vi "sub vi - temperature delay v2.vi"(10 "temp values IN":T1, 11 "temp signals":T2) -> (0 "T2-N":dbl, 1 "T2-L":dbl, 2 "T1-N":dbl, 3 "T1-L":dbl, 4 "temp values OUT":T1)   [LabVIEW 2013]
uses:
  program files/Global 1.vi
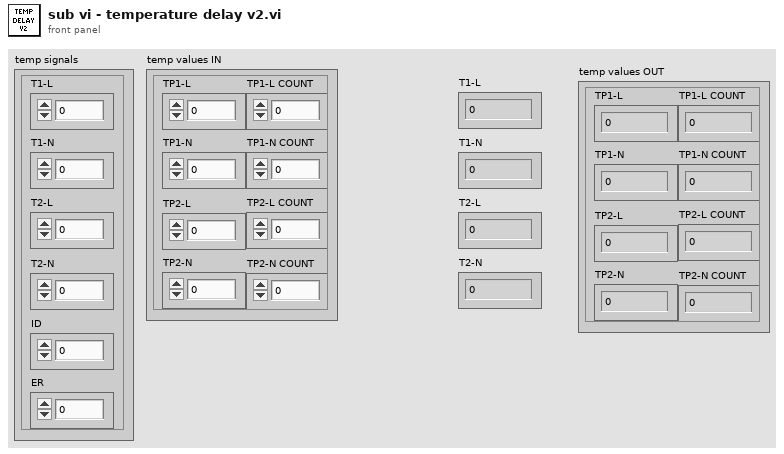
[diagram p1: front panel]
types:
  T1 = cluster{"TP1-L":dbl, "TP1-N":dbl, "TP2-L":dbl, "TP2-N":dbl, "TP1-L COUNT":dbl, "TP1-N COUNT":dbl, "TP2-L COUNT":dbl, "TP2-N COUNT":dbl}
  T2 = cluster{"T1-L":dbl, "T1-N":dbl, "T2-L":dbl, "T2-N":dbl, "ID":dbl, "ER":dbl}
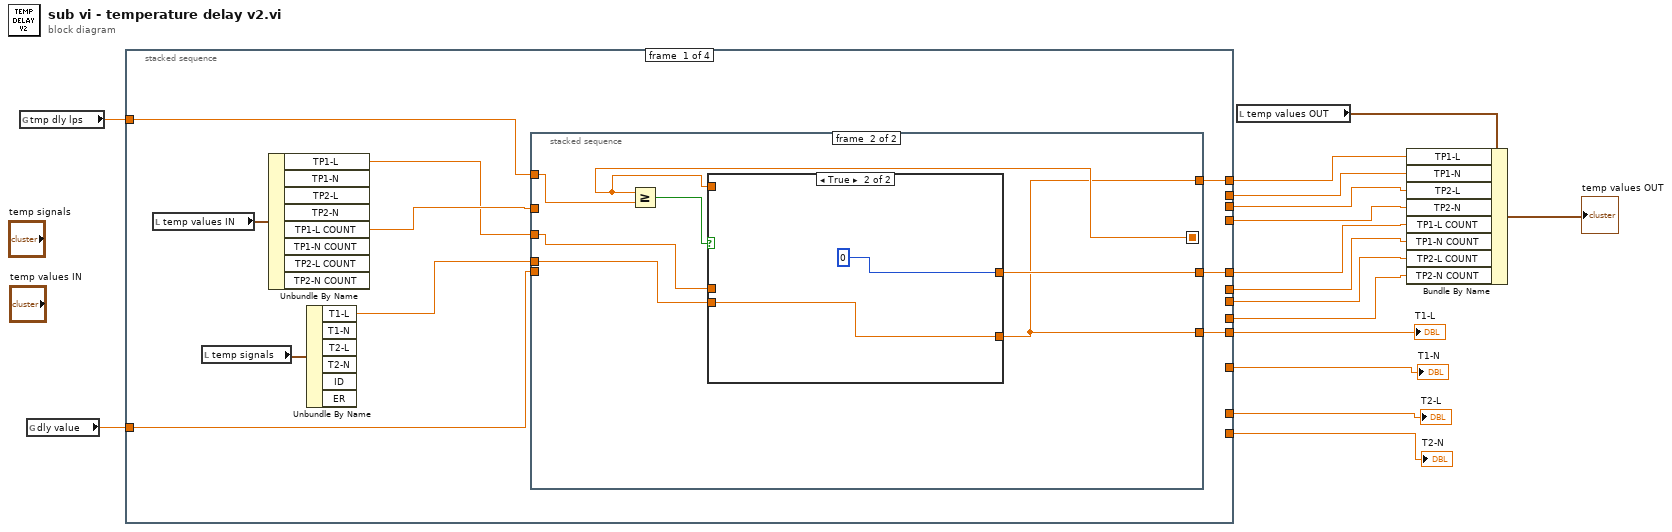
[diagram p0: block diagram]
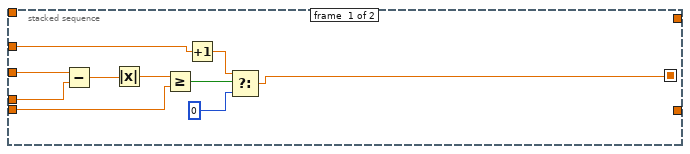
[diagram p2: hidden frame]
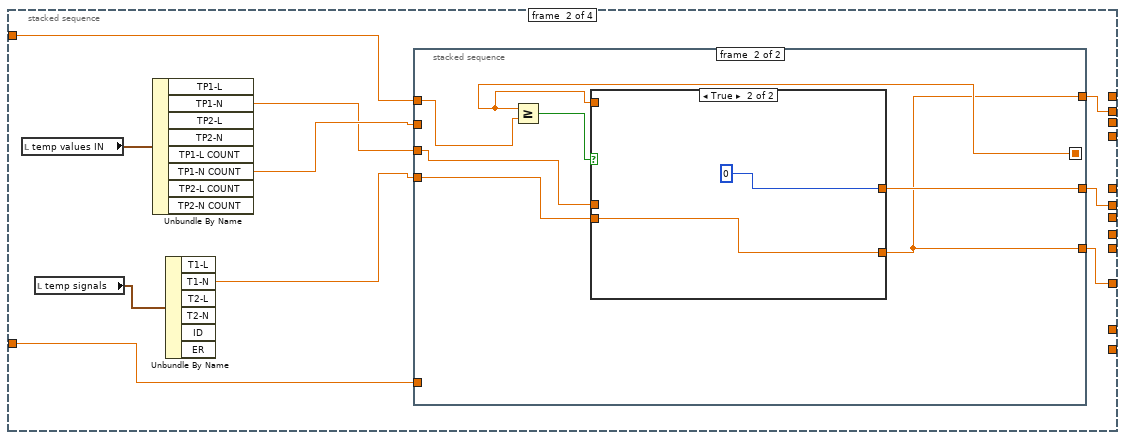
[diagram p4: hidden frame]
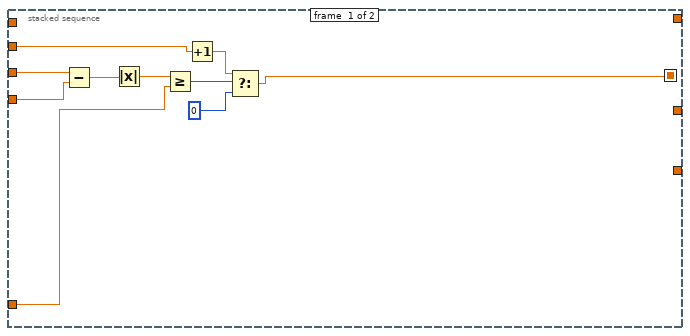
[diagram p5: hidden frame]
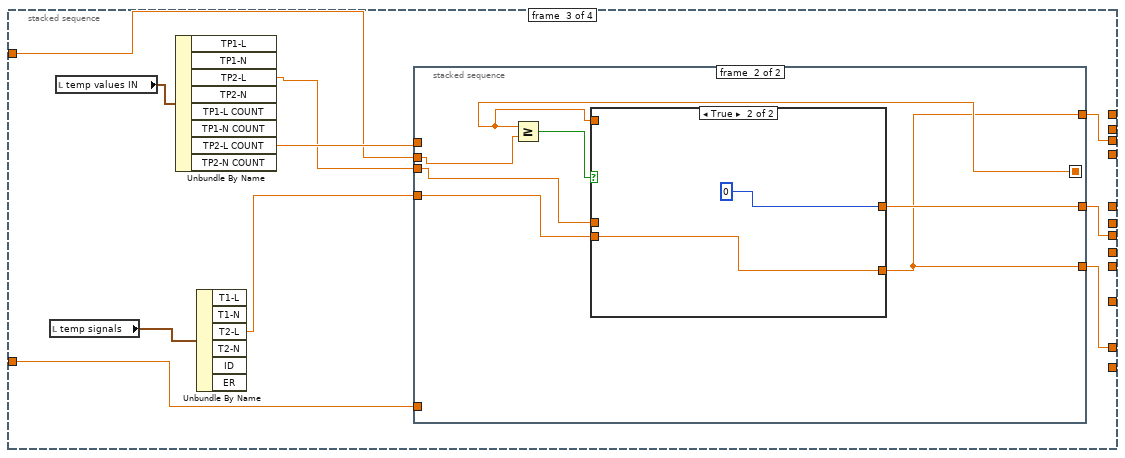
[diagram p7: hidden frame]
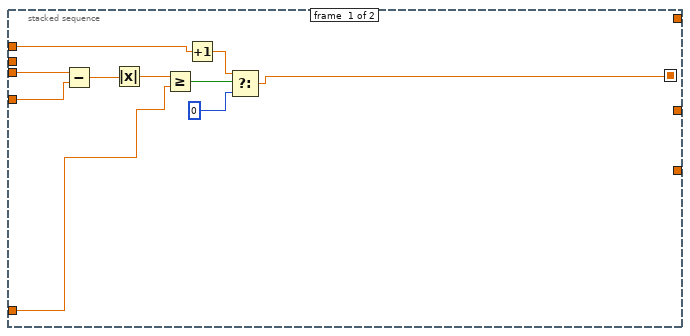
[diagram p8: hidden frame]
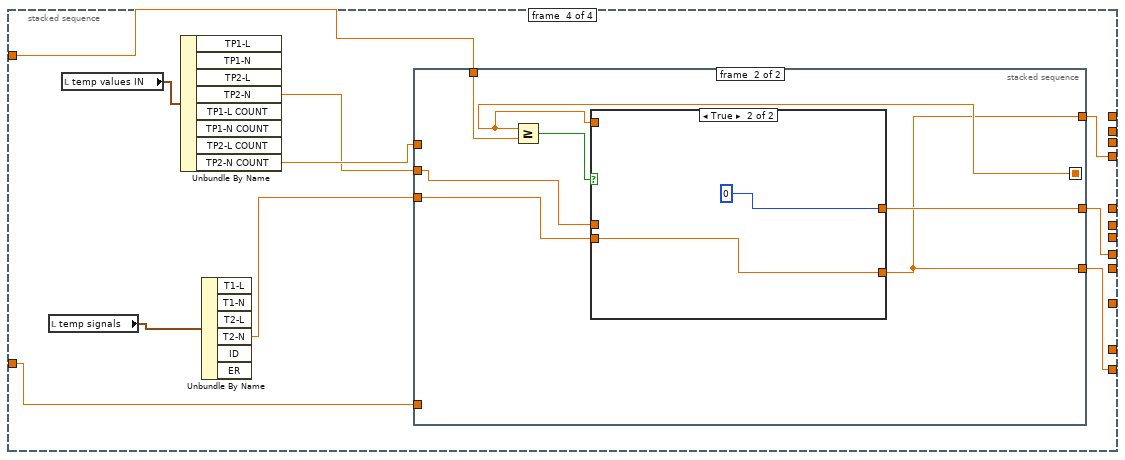
[diagram p10: hidden frame]
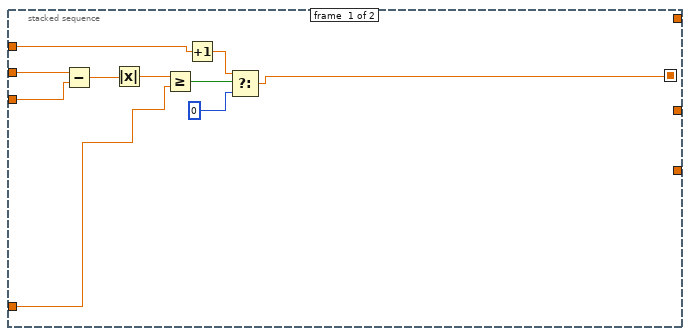
[diagram p11: hidden frame]
diagram:
  n1 = global read "Global 1.vi" "tmp dly lps"() -> (w2:dbl)
  n2 = global read "Global 1.vi" "dly value"() -> (w1:dbl)
  n3 = stacked-sequence {
    tunnel: [w26 _ _ _] -> w14
    tunnel: [w25 _ _ _] -> w13
    tunnel: [w24 _ _ _] -> w12
    tunnel: [_ w57 _ _] -> w11
    tunnel: [_ w56 _ _] -> w10
    tunnel: [_ w55 _ _] -> w9
    tunnel: [_ _ w88 _] -> w8
    tunnel: [_ _ w87 _] -> w7
    tunnel: [_ _ w86 _] -> w6
    tunnel: [_ _ _ w119] -> w5
    tunnel: [_ _ _ w118] -> w4
    tunnel: [_ _ _ w117] -> w3
    tunnel: w2 -> [w18 w48 w79 w110]
    tunnel: w1 -> [w17 w49 w80 w111]
    frame #0 {
      n4 = local read "temp values IN"() -> (w22:T1)
      n5 = local read "temp signals"() -> (w23:T2)
      n6 = Unbundle By Name(w22) -> ("TP1-L"=w20:dbl, "TP1-L COUNT"=w21:dbl)  [unwired: 6 out]
      n7 = Unbundle By Name(w23) -> ("T1-L"=w19:dbl)  [unwired: 5 out]
      n8 = stacked-sequence {
        seq-local: [w28 _] -> [_ w39]
        tunnel: w20 -> [w31 w41]
        tunnel: w19 -> [w30 w42]
        tunnel: w21 -> [w29 _]
        tunnel: [_ w40] -> w26
        tunnel: [_ w38] -> w25
        tunnel: [_ w38] -> w24
        tunnel: w17 -> [w27 _]
        tunnel: w18 -> [_ w37]
        frame #0 {
          n9 = Subtract(x=w31, y=w30) -> (x-y=w36:dbl)
          n10 = Absolute Value(x=w36) -> (abs(x)=w35:dbl)
          n11 = Greater Or Equal?(x=w35, y=w27) -> (x >= y?=w34:bool)
          n12 = Increment(x=w29) -> (x+1=w33:dbl)
          n13 = Select(t=w33, s=w34, f=0) -> (s? t:f=w28:dbl)
        }
        frame #1 {
          n14 = Greater Or Equal?(x=w39, y=w37) -> (x >= y?=w43:bool)
          n15 = case shown="True" w43 {
            tunnel: [w45 w47] -> w38
            tunnel: w42 -> [_ w47]
            tunnel: w41 -> [w45 _]
            tunnel: [w44 0] -> w40
            tunnel: w39 -> [w44 _]
            frame False {
            }
            frame True {
            }
          }
        }
      }
    }
    frame #1 {
      n16 = local read "temp values IN"() -> (w54:T1)
      n17 = local read "temp signals"() -> (w51:T2)
      n18 = Unbundle By Name(w54) -> ("TP1-N"=w52:dbl, "TP1-N COUNT"=w53:dbl)  [unwired: 6 out]
      n19 = Unbundle By Name(w51) -> ("T1-N"=w50:dbl)  [unwired: 5 out]
      n20 = stacked-sequence {
        seq-local: [w59 _] -> [_ w70]
        tunnel: w52 -> [w62 w72]
        tunnel: w50 -> [w61 w73]
        tunnel: w53 -> [w60 _]
        tunnel: [_ w71] -> w56
        tunnel: [_ w69] -> w57
        tunnel: [_ w69] -> w55
        tunnel: w49 -> [w58 _]
        tunnel: w48 -> [_ w68]
        frame #0 {
          n21 = Subtract(x=w62, y=w61) -> (x-y=w67:dbl)
          n22 = Absolute Value(x=w67) -> (abs(x)=w66:dbl)
          n23 = Greater Or Equal?(x=w66, y=w58) -> (x >= y?=w65:bool)
          n24 = Increment(x=w60) -> (x+1=w64:dbl)
          n25 = Select(t=w64, s=w65, f=0) -> (s? t:f=w59:dbl)
        }
        frame #1 {
          n26 = Greater Or Equal?(x=w70, y=w68) -> (x >= y?=w74:bool)
          n27 = case shown="True" w74 {
            tunnel: [w76 w78] -> w69
            tunnel: w73 -> [_ w78]
            tunnel: w72 -> [w76 _]
            tunnel: [w75 0] -> w71
            tunnel: w70 -> [w75 _]
            frame False {
            }
            frame True {
            }
          }
        }
      }
    }
    frame #2 {
      n28 = local read "temp signals"() -> (w84:T2)
      n29 = local read "temp values IN"() -> (w85:T1)
      n30 = Unbundle By Name(w85) -> ("TP2-L"=w82:dbl, "TP2-L COUNT"=w83:dbl)  [unwired: 6 out]
      n31 = Unbundle By Name(w84) -> ("T2-L"=w81:dbl)  [unwired: 5 out]
      n32 = stacked-sequence {
        seq-local: [w90 _] -> [_ w101]
        tunnel: w82 -> [w93 w103]
        tunnel: w81 -> [w92 w104]
        tunnel: w83 -> [w91 _]
        tunnel: [_ w102] -> w87
        tunnel: [_ w100] -> w88
        tunnel: [_ w100] -> w86
        tunnel: w80 -> [w89 _]
        tunnel: w79 -> [_ w99]
        frame #0 {
          n33 = Subtract(x=w93, y=w92) -> (x-y=w98:dbl)
          n34 = Absolute Value(x=w98) -> (abs(x)=w97:dbl)
          n35 = Greater Or Equal?(x=w97, y=w89) -> (x >= y?=w96:bool)
          n36 = Increment(x=w91) -> (x+1=w95:dbl)
          n37 = Select(t=w95, s=w96, f=0) -> (s? t:f=w90:dbl)
        }
        frame #1 {
          n38 = Greater Or Equal?(x=w101, y=w99) -> (x >= y?=w105:bool)
          n39 = case shown="True" w105 {
            tunnel: [w107 w109] -> w100
            tunnel: w104 -> [_ w109]
            tunnel: w103 -> [w107 _]
            tunnel: [w106 0] -> w102
            tunnel: w101 -> [w106 _]
            frame False {
            }
            frame True {
            }
          }
        }
      }
    }
    frame #3 {
      n40 = local read "temp signals"() -> (w116:T2)
      n41 = local read "temp values IN"() -> (w115:T1)
      n42 = Unbundle By Name(w115) -> ("TP2-N"=w113:dbl, "TP2-N COUNT"=w114:dbl)  [unwired: 6 out]
      n43 = Unbundle By Name(w116) -> ("T2-N"=w112:dbl)  [unwired: 5 out]
      n44 = stacked-sequence {
        seq-local: [w121 _] -> [_ w132]
        tunnel: w113 -> [w124 w134]
        tunnel: w112 -> [w123 w135]
        tunnel: w114 -> [w122 _]
        tunnel: [_ w133] -> w118
        tunnel: [_ w131] -> w119
        tunnel: [_ w131] -> w117
        tunnel: w111 -> [w120 _]
        tunnel: w110 -> [_ w130]
        frame #0 {
          n45 = Subtract(x=w124, y=w123) -> (x-y=w129:dbl)
          n46 = Absolute Value(x=w129) -> (abs(x)=w128:dbl)
          n47 = Greater Or Equal?(x=w128, y=w120) -> (x >= y?=w127:bool)
          n48 = Increment(x=w122) -> (x+1=w126:dbl)
          n49 = Select(t=w126, s=w127, f=0) -> (s? t:f=w121:dbl)
        }
        frame #1 {
          n50 = Greater Or Equal?(x=w132, y=w130) -> (x >= y?=w136:bool)
          n51 = case shown="True" w136 {
            tunnel: [w138 w140] -> w131
            tunnel: w135 -> [_ w140]
            tunnel: w134 -> [w138 _]
            tunnel: [w137 0] -> w133
            tunnel: w132 -> [w137 _]
            frame False {
            }
            frame True {
            }
          }
        }
      }
    }
  }
  "T1-N" <- w9
  "T2-L" <- w6
  "T2-N" <- w3
  "T1-L" <- w12
  n52 = local read "temp values OUT"() -> (w16:T1)
  n53 = Bundle By Name(cluster=w16, "TP1-L"=w13, "TP1-N"=w11, "TP2-L"=w8, "TP2-N"=w5, "TP1-L COUNT"=w14, "TP1-N COUNT"=w10, "TP2-L COUNT"=w7, "TP2-N COUNT"=w4) -> (→"temp values OUT":T1)
